vi "practica1_2.3.vi"() -> ()   [LabVIEW 2016]
panel:
  out "END":bool
  out "Thermometer":dbl(slide) scale=25.0..90.0
  out "Tank":dbl(slide) scale=0.0..10.0
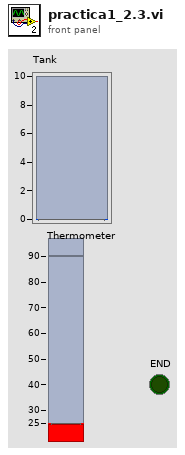
[diagram p1: front panel]
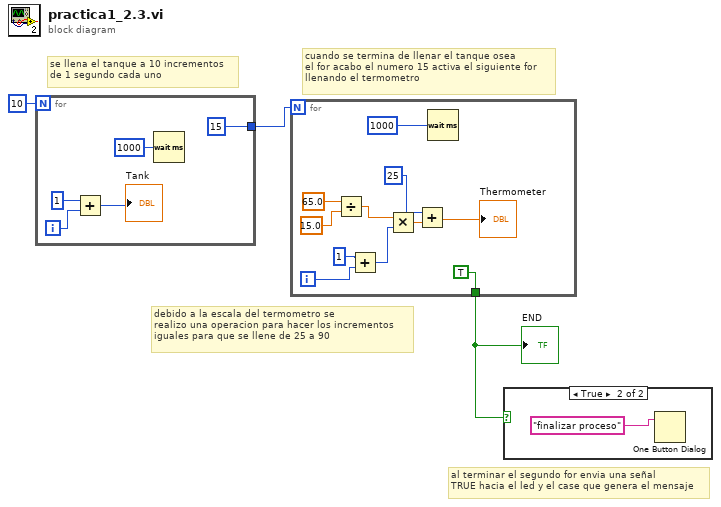
[diagram p0: block diagram]
diagram:
  # "al terminar el segundo for envia una señal\nTRUE hacia el led y el case que genera el mensaje"
  # "debido a la escala del termometro se \nrealizo una operacion para hacer los incrementos\niguales para que se llene de 25 a 90"
  # "cuando se termina de llenar el tanque osea \nel for acabo el numero 15 activa el siguiente for\nllenando el termometro"
  # "se llena el tanque a 10 incrementos \nde 1 segundo cada uno"
  n1 = for {
    N: 10 -> [_]
    tunnel: [15] -> w2
    i -> [w7]
    n2 = Add(x=1, y=w7) -> (x+y=→"Tank":i32)
    n3 = Wait (ms)(milliseconds to wait=u32 1000) -> ()  [unwired: 1 out]
  }
  n4 = for {
    N: w2 -> [_]
    tunnel: [TRUE] -> w1
    i -> [w9]
    n5 = Divide(x=65.0, y=15.0) -> (x/y=w16:dbl)
    n6 = Add(x=1, y=w9) -> (x+y=w11:i32)
    n7 = Multiply(x=w16, y=w11) -> (x*y=w13:dbl)
    n8 = Add(x=25, y=w13) -> (x+y=→"Thermometer":dbl)
    n9 = Wait (ms)(milliseconds to wait=u32 1000) -> ()  [unwired: 1 out]
  }
  "END" <- w1
  n10 = case shown="True" w1 {
    frame False {
    }
    frame True {
      n11 = One Button Dialog(message="finalizar proceso") -> ()  [unwired: 1 in, 1 out]
    }
  }
